vi "Previous x cam data.vi"() -> ()   [LabVIEW 2016]
panel:
  out "L457 X V41U3":dbl
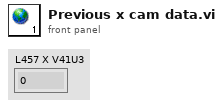
[diagram p1: front panel]
diagram:
